vi "DAQmx Create Channel (AI-Sound Pressure-Microphone).vi"(0 "task in":refnum<k21>, 1 "maximum sound pressure level":dbl=100.0 format="%0.2f", 3 "input terminal configuration":i32(ring)=-1 items=["default"=-1, "RSE"=10083, "NRSE"=10078, "Differential"=10106, "Pseudodifferential"=12529], 5 "physical channels":tag, 6 "current excitation source":i32(ring)=10200 items=["Internal"=10200, "External"=10167, "None"=10230], 7 "name to assign":string, 8 "current excitation value":dbl=0.004, 9 "units":i32(ring)=10081 items=["Pascals"=10081, "From Custom Scale"=10065], 11 "error in":errorcluster, 12 "custom scale name":tag, 13 "microphone sensitivity":dbl=10.0) -> (4 "task out":refnum<k21>, 15 "error out":errorcluster)   [LabVIEW 2013]
doc: "Creates channel(s) that use a microphone to measure sound pressure."
uses:
  C:/Program Files (x86)/National Instruments/LabVIEW 2013/resource/objmgr/daqmx.rc
panel:
  # "input limits"
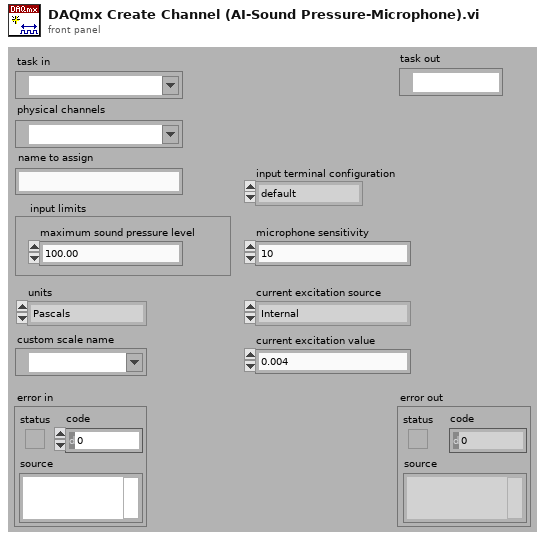
[diagram p1: front panel]
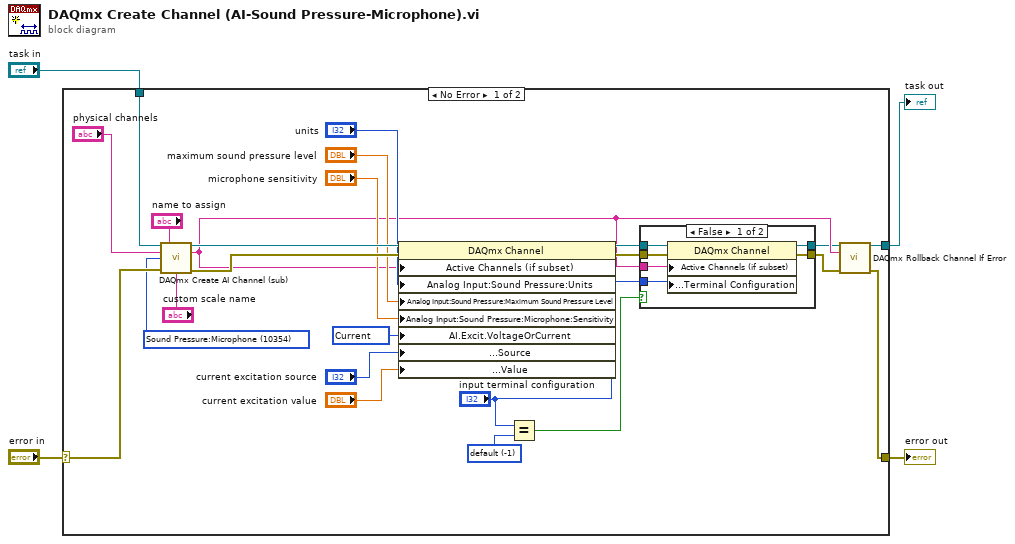
[diagram p0: block diagram]
diagram:
  n1 = case shown="No Error" "error in" {
    selector: "error in" -> [w26 w38]
    tunnel: [w20 w38] -> w2
    tunnel: "task in" -> [w27 w37]
    tunnel: [w21 w37] -> w1
    frame No Error {
      w5 = 10134 items=["Voltage"=10322, "Current"=10134] ("AI.Excit.VoltageOrCurrent")
      w10 = -1 items=["default"=-1, "differential"=10106, "RSE"=10083, "NRSE"=10078] ("input terminal configuration")
      w16 = 10354 items=["Voltage"=10322, "Current"=10134, "More:Voltage:Custom with Excitation"=10323, "More:Current:Custom with Excitation"=10136, "Frequency"=10181, "Period"=10257, "Resistance"=10278, "Temperature:Thermocouple"=10303, "Temperature:Thermistor"=10302, "Temperature:RTD"=10301, "Temperature:Built-in Sensor"=10311, "Strain Gage"=10300, "LVDT"=10352, "RVDT"=10353, "Accelerometer:Voltage Input"=10355, "Accelerometer:Current Input"=10356, "Sound Pressure:Microphone"=10354] ("measurement type")
      n2 = call "DAQmx Create AI Channel (sub).vi"("task in"=w27, "virtual channel name"="name to assign", "physical channel name"="physical channels", "measurement type"=w16, "error in"=w26, "custom scale"="custom scale name") -> ("task out"=w28:refnum<k21>, "channel names"=w11:string, "error out"=w23:errorcluster)  [unwired: 1 in, 6 out]
      n3 = property class="DAQmx Channel"(reference=w28, error in=w23, "Active Channels (if subset)"=w11, "Analog Input:Sound Pressure:Units"="units", "Analog Input:Sound Pressure:Maximum Sound Pressure Level"="maximum sound pressure level", "Analog Input:Sound Pressure:Microphone:Sensitivity"="microphone sensitivity", "AI.Excit.VoltageOrCurrent"=w5, "Analog Input:General Properties:Signal Conditioning:Excitation:Source"="current excitation source", "Analog Input:General Properties:Signal Conditioning:Excitation:Value"="current excitation value") -> (reference out=w13:refnum<k21>, error out=w12:errorcluster)
      n4 = Equal?(x="input terminal configuration", y=w10) -> (x = y?=w9:bool)
      n5 = case shown="False" w9 {
        tunnel: w12 -> [w34 w36]
        tunnel: [w33 w35] -> w7
        tunnel: [w32 w36] -> w6
        tunnel: "input terminal configuration" -> [w31 _]
        tunnel: w11 -> [w30 _]
        tunnel: w13 -> [w29 w35]
        frame False {
          n6 = property class="DAQmx Channel"(reference=w29, error in=w34, "Active Channels (if subset)"=w30, "Analog Input:General Properties:Input Configuration:Terminal Configuration"=w31) -> (reference out=w33:refnum<k21>, error out=w32:errorcluster)
        }
        frame True {
        }
      }
      n7 = call "DAQmx Rollback Channel If Error.vi"("task in"=w7, "channel names"=w11, "error in"=w6) -> ("task out"=w21:refnum<k21>, "error out"=w20:errorcluster)  [unwired: 11 out]
    }
    frame Error {
    }
  }
  "error out" <- w2
  "task out" <- w1
